vi "Read UI Info From Configuration.vi"(8 "error in (no error)":errorcluster, 11 "node in":refnum<class "RIO Target.lvclass">) -> (0 "error out":errorcluster, 1 "CLIP XML Path":path, 2 "Input Paths":T1={"Golden Template (Source) - (make relative)"=path "E:/Documents/Projects/SPIAPI/Scripting Code  with State Machine 01_12_15 - IO Node Control Still Needs Updating/IONode", "Destination Generated Code (make relative)"=path "E:/Documents/Projects/SPIAPI/Examples", "LabVIEW Project to Script"=path "E:/Documents/Projects/SPIAPI/Examples/SPI Engine Example.lvproj", "Placement VI"=path "E:/Documents/Projects/SPIAPI/Examples/PMOD Example(FPGA).vi"}, 3 "node out":refnum<class "RIO Target.lvclass">)   [LabVIEW 2014, in "RIO Target.lvclass"]
uses:
  RIO Target.lvclass
  Scripting/Initialization Scripting/State Machine/Controls/Input Paths.ctl
  RIO Target.lvclass/RIO Target.ctl
  RIO Target Configuration/RIO Target Configuration.lvclass/RIO Target Configuration.ctl
  RIO Target Configuration/RIO Target Configuration.lvclass
  Scripting/Initialization Scripting/SPI Engine Scripting.lvlib
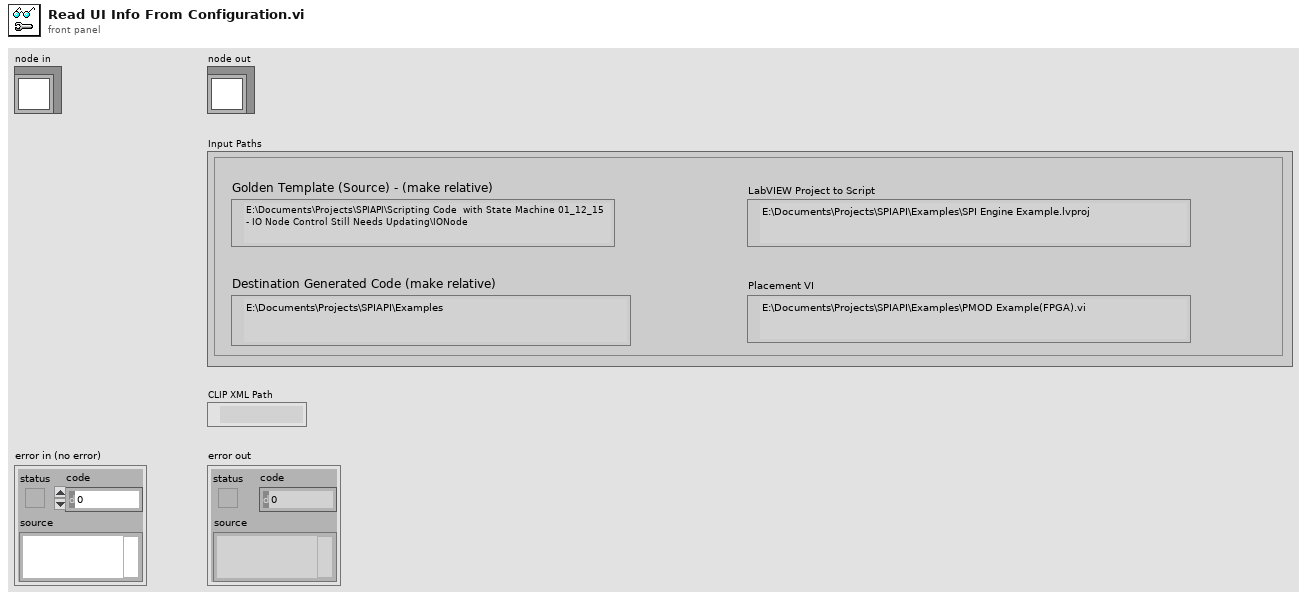
[diagram p1: front panel]
types:
  T1 = typedef "SPI Engine Scripting.lvlib/Input Paths.ctl" = cluster{"Golden Template (Source) - (make relative)":path, "Destination Generated Code (make relative)":path, "LabVIEW Project to Script":path, "Placement VI":path}
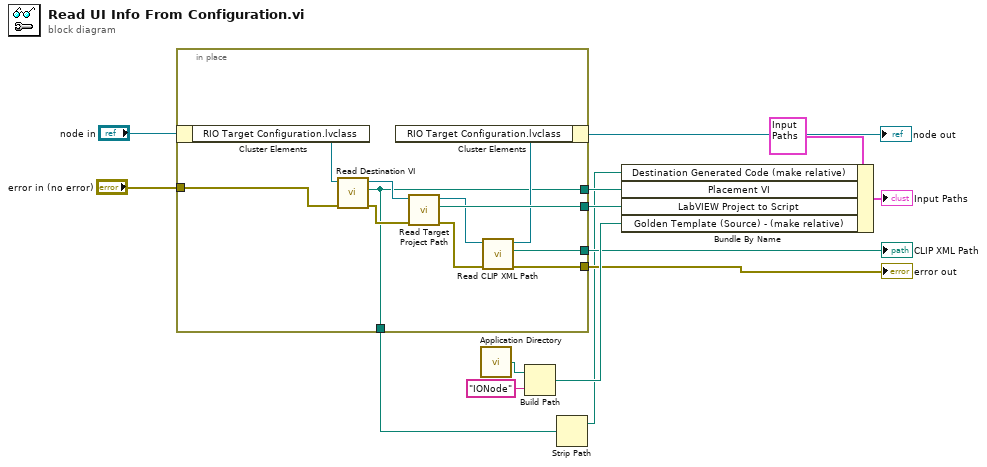
[diagram p0: block diagram]
diagram:
  n1 = in-place {
    in-place-border: [w15] -> w8
    in-place-border: [w24] -> w7
    in-place-border: "error in (no error)" -> [w17]
    in-place-border: [w19] -> w5
    in-place-border: [w18] -> w3
    in-place-border: [w15] -> w2
    n2 = in-place-cluster #1("node in") -> ("RIO Target Configuration.lvclass"=w16:refnum<class "RIO Target Configuration.lvclass">)
    n3 = call "Read Destination VI.vi"("error in (no error)"=w17, "RIO Target Configuration in"=w16) -> ("error out"=w23:errorcluster, "Destination VI"=w15:path, "RIO Target Configuration out"=w25:refnum<class "RIO Target Configuration.lvclass">)  [unwired: 7 in]
    n4 = call "Read Target Project Path.vi"("error in (no error)"=w23, "RIO Target Configuration in"=w25) -> ("error out"=w22:errorcluster, "Target Project Path"=w24:path, "RIO Target Configuration out"=w21:refnum<class "RIO Target Configuration.lvclass">)  [unwired: 7 in]
    n5 = call "Read CLIP XML Path.vi"("error in (no error)"=w22, "RIO Target Configuration in"=w21) -> ("error out"=w19:errorcluster, "CLIP XML Path"=w18:path, "RIO Target Configuration out"=w20:refnum<class "RIO Target Configuration.lvclass">)  [unwired: 7 in]
    n6 = in-place-cluster #1("RIO Target Configuration.lvclass"=w20) -> (→"node out":refnum<class "RIO Target.lvclass">)
  }
  "error out" <- w5
  "CLIP XML Path" <- w3
  n7 = call <vilib>:"Application Directory.vi"() -> ("Application Directory"=w11:path)
  n8 = Build Path(base path=w11, name or relative path="IONode") -> (appended path=w9:path)
  n9 = Strip Path(path=w2) -> (stripped path=w1:path)  [unwired: 1 out]
  n10 = Bundle By Name(cluster=T1 {"Golden Template (Source) - (make relative)"=path "C:/Users/iknox/Documents/Configuration Editor Sandbox/IONode", "Destination Generated Code (make relative)"=path "C:/Users/iknox/Desktop/Test", "LabVIEW Project to Script"=path "C:/Users/iknox/Desktop/Untitled Project 1.lvproj", "Placement VI"=path "C:/Users/iknox/Desktop/Untitled 3.vi"} ("Input Paths"), "Destination Generated Code (make relative)"=w1, "Placement VI"=w8, "LabVIEW Project to Script"=w7, "Golden Template (Source) - (make relative)"=w9) -> (→"Input Paths":T1)
